vi "ACQ Read.vi"(8 "error in (no error)":errorcluster, 11 "AD4212C in":refnum<class "AD4212C.lvclass">) -> (0 "error out":errorcluster, 3 "AD4212C out":refnum<class "AD4212C.lvclass">)   [LabVIEW 2014, in "AD4212C.lvlib" / "AD4212C.lvclass"]
doc: "Lee los datos del Buffer, detecta errores e inestabilidades de la adquisición. Convierte los datos a formato SGL."
uses:
  AD4212C.lvclass
  AD4212C.lvclass/AD4212C.ctl
  API/AD4212C Lib.lvlib
  DriverMasterAsync/builds/DriverMasterAsync.lvlibp/Modules/HAL/DriverMasterAsync/DriverMasterAsyncClass/DriverMasterAsync.lvclass
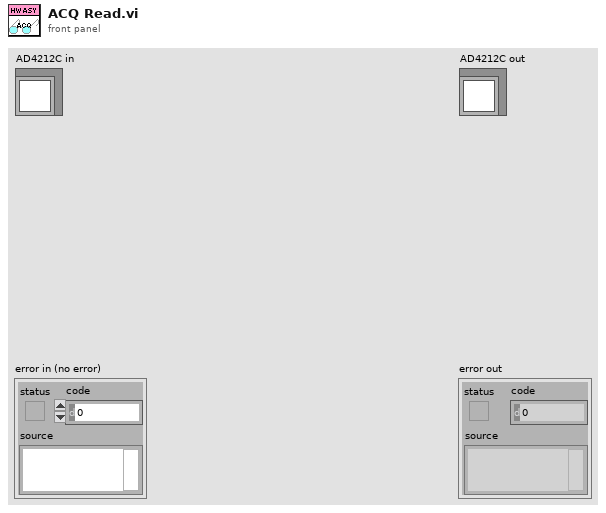
[diagram p1: front panel]
types:
  T1 = typedef "AD4212C Lib.lvlib/Connection Data.ctl" = cluster{"Conection Data":refnum<visa-resource-name>}
  T2 = typedef "DriverMasterAsync.lvlibp/WINFAS 2 Data Queue.lvlib/Async Acquisition Data Cluster.ctl" = cluster{"Data":sgl[]}
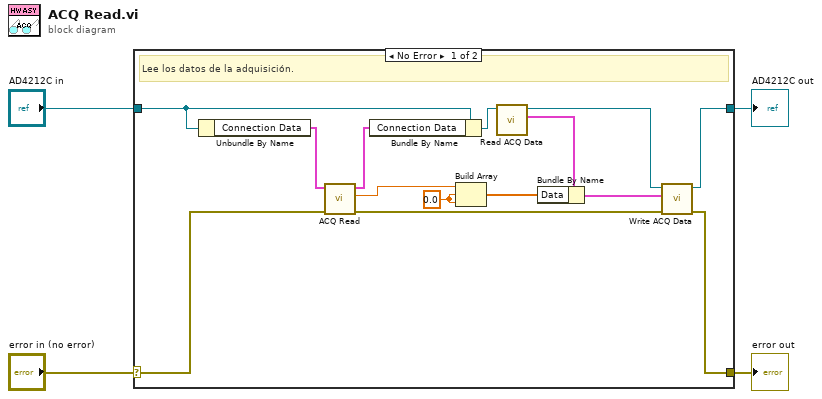
[diagram p0: block diagram]
diagram:
  n1 = case shown="No Error" "error in (no error)" {
    selector: "error in (no error)" -> [w14 w20]
    tunnel: [w12 w20] -> w3
    tunnel: [w18 w19] -> w1
    tunnel: "AD4212C in" -> [w15 w19]
    frame No Error {
      w8 = sgl 0.0 ("element")
      # "Lee los datos de la adquisición."
      n2 = Unbundle By Name(w15) -> ("Connection Data"=w17:T1)
      n3 = call "ACQ Read.vi"("error in (no error)"=w14, "VISA resource name In"=w17) -> ("error out"=w13:errorcluster, "Value"=w5:sgl, "VISA resource name Out"=w16:T1)  [unwired: 7 in]
      n4 = Bundle By Name(cluster=w15, "Connection Data"=w16) -> (w11:refnum<class "AD4212C.lvclass">)
      n5 = Build Array(w5, w8, w8) -> (w7:sgl[])
      n6 = call "Read ACQ Data.vi"("DriverMasterAsync in"=w11) -> ("ACQ Data"=w9:T2, "DriverMasterAsync out"=w10:refnum<class "AD4212C.lvclass">)  [unwired: 8 in, 1 out]
      n7 = Bundle By Name(cluster=w9, "Data"=w7) -> (w6:T2)
      n8 = call "Write ACQ Data.vi"("error in (no error)"=w13, "ACQ Data"=w6, "DriverMasterAsync in"=w10) -> ("error out"=w12:errorcluster, "DriverMasterAsync out"=w18:refnum<class "AD4212C.lvclass">)  [unwired: 7 in]
    }
    frame Error {
    }
  }
  "error out" <- w3
  "AD4212C out" <- w1
